vi "Add Timestamp to String.vi"(1 "String In":string, 12 "Add (T)":bool=TRUE) -> (21 "String Out":string)   [LabVIEW 2017]
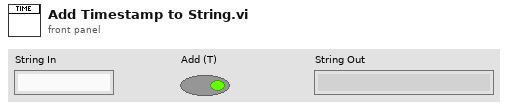
[diagram p1: front panel]
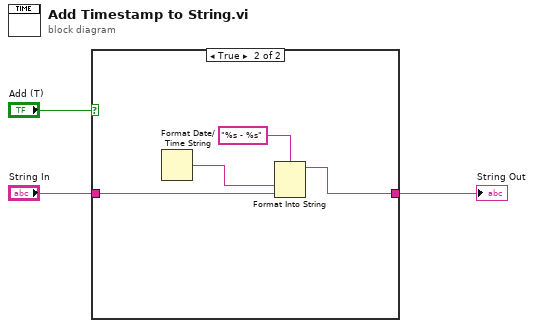
[diagram p0: block diagram]
diagram:
  n1 = case shown="True" "Add (T)" {
    tunnel: [w4 w5] -> w2
    tunnel: "String In" -> [w4 w8]
    frame False {
    }
    frame True {
      n2 = Format Date/Time String() -> (date/time string=w7:string)  [unwired: 3 in]
      n3 = Format Into String(format string="%s - %s", w7, w8) -> (resulting string=w5:string)  [unwired: 2 in, 1 out]
    }
  }
  "String Out" <- w2
